vi "Assemble Car Wash Display ViewManager.vi"(9 "Active Station Time Remaining View":refnum<class "Active Option Elapsed Time View Definition.lvclass">, 10 "Active Station View":refnum<class "Active Option View Definition.lvclass">, 11 "Car Wash Status View":refnum<class "Car Wash Status View Definition.lvclass">) -> (3 "Car Wash Display ViewManager out":refnum<class "Car Wash Display ViewManager.lvclass">)   [LabVIEW 2019, in "Car Wash Display ViewManager.lvclass"]
uses:
  <vilib>/gpm_packages/@cs/Car-wash/Source/Car Wash Display ViewManager/Car Wash Display ViewManager/Car Wash Display ViewManager.lvclass
  C:/Program Files/National Instruments/LabVIEW 2019/vi.lib/gpm_packages/@cs/mva-viewable/Source/IViewManager/IViewManager/IViewManager.lvclass
  <vilib>/gpm_packages/@cs/Car-wash/Source/Car Wash Status View Definition/Car Wash Status View Definition/Car Wash Status View Definition.lvclass
  C:/Program Files/National Instruments/LabVIEW 2019/vi.lib/gpm_packages/@cs/mva-viewable/Source/IViewable/IViewable/IViewable.lvclass
  <vilib>/gpm_packages/@cs/Car-wash/Source/Active Station View Definition/Active Station View Definition/Active Option View Definition.lvclass
  <vilib>/gpm_packages/@cs/Car-wash/Source/Active Station Time Remaining View Definition/Active Station Time Remaining View Definition/Active Option Elapsed Time View Definition.lvclass
  <vilib>/gpm_packages/@cs/mva-viewable/Source/IViewManager/IViewManager Messages/Launch Nested Views Msg/Launch Nested Views Msg.lvclass/Launch Nested Views Msg.ctl
  <vilib>/gpm_packages/@cs/mva-viewable/Source/IViewManager/IViewManager/IViewManager.lvclass/IViewManager.ctl
  <vilib>/gpm_packages/@cs/mva-viewable/Source/IViewManager/IViewManager Messages/Launch Nested Views Msg/Pack Launch Nested Views Msg.vi
  <vilib>/gpm_packages/@cs/mva-viewable/Source/IViewManager/IViewManager Messages/Launch Nested Views Msg/Launch Nested Views Msg.lvclass
  <vilib>/gpm_packages/@cs/mva-viewable/Source/IViewManager/IViewManager/IViewManager.lvclass
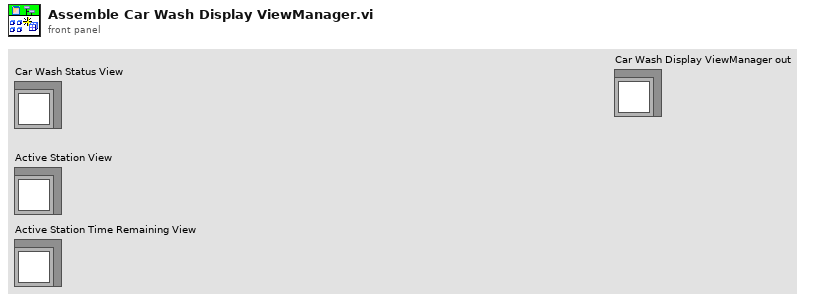
[diagram p1: front panel]
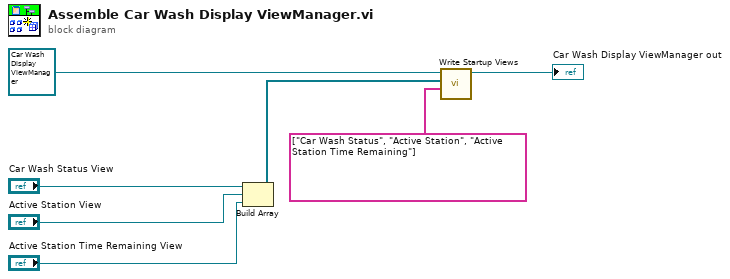
[diagram p0: block diagram]
diagram:
  n1 = Build Array("Car Wash Status View", "Active Station View", "Active Station Time Remaining View") -> (w6:refnum<class "IViewable.lvclass">[])
  n2 = call <vilib>:"Write Startup Views.vi"("View Labels"=string[] ["Car Wash Status", "Active Station", "Active Station Time Remaining"], "Startup Views"=w6, "IViewManager in"=refnum<class "Car Wash Display ViewManager.lvclass"> refnum ("Car Wash Display ViewManager.lvlib:Car Wash Display ViewManager.lvclass")) -> ("IViewManager out"=→"Car Wash Display ViewManager out":refnum<class "Car Wash Display ViewManager.lvclass">)  [unwired: 8 in]
